vi "Temperature Change Conversion.vi"(9 "Current Wavelength (0 nm)":dbl format="%#_10g", 10 "Nominal Wavelength (0 nm)":dbl format="%#_10g") -> (2 "Temperature Change (°C)":dbl)   [LabVIEW 2015, in "Micron Optics sm130.lvlib"]
doc: "Converts the waveform shift to temperature change value in celcius.\n\n<b>Note:</b>\n1.) This conversion VI is compatible with Micron Optics sensor model os4100."
uses:
  Micron Optics sm130.lvlib
panel:
  # "This conversion VI is compatible with Micron Optics sensor model os4100."
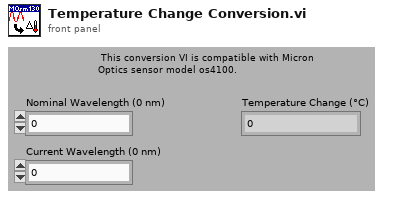
[diagram p1: front panel]
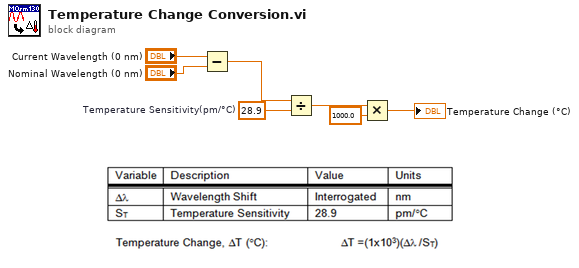
[diagram p0: block diagram]
diagram:
  w4 = 28.9  # Temperature Sensitivity(pm/°C)
  n1 = Subtract(x="Current Wavelength (0 nm)", y="Nominal Wavelength (0 nm)") -> (x-y=w5:dbl)
  n2 = Divide(x=w5, y=w4) -> (x/y=w3:dbl)
  n3 = Multiply(x=w3, y=1000.0) -> (x*y=→"Temperature Change (°C)":dbl)
